vi "Set Stop Trigger (Log Indefinitely).vi"(8 "error in (no error)":errorcluster, 11 "Data Logging Specification Ref in":T1) -> (0 "error out":errorcluster, 3 "Data Logging Specification Ref out":T1)   [LabVIEW 2020, in "NI_VS Data Logging API.lvlib"]
doc: "Specifies a trigger condition on which to stop logging data. You also can specify whether to continue logging channel data for a set period of time after the trigger condition occurs.\n\nYou must manually select the polymorphic instance to use."
uses:
  <vilib>/NI VeriStand/Execution/DataLogging/NI_VS Data Logging API.lvlib
  <vilib>/NI VeriStand/Execution/DataLogging/DataLoggingSpecification Ref.ctl
  NationalInstruments.VeriStand.ClientAPI
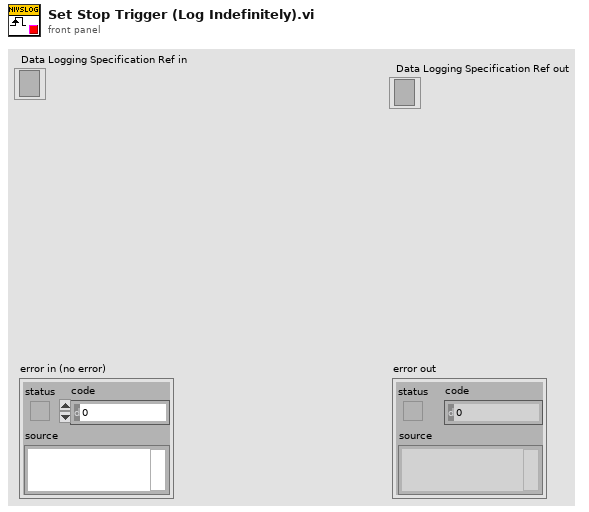
[diagram p1: front panel]
types:
  T1 = typedef "NI_VS Data Logging API.lvlib/DataLoggingSpecification Ref.ctl" = refnum<k24>
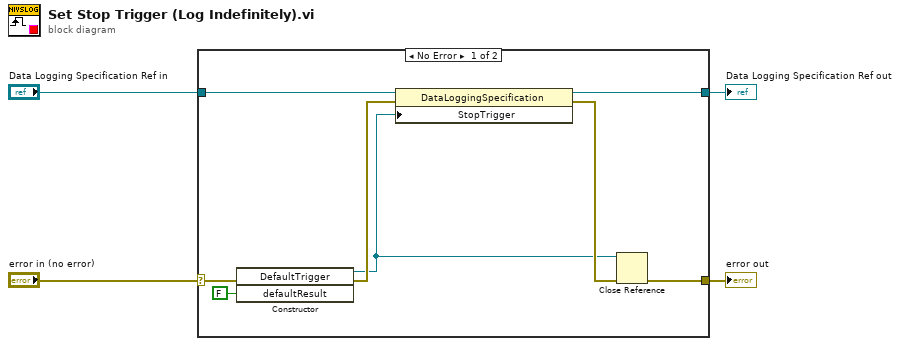
[diagram p0: block diagram]
diagram:
  n1 = case shown="No Error" "error in (no error)" {
    selector: "error in (no error)" -> [w9 w14]
    tunnel: "Data Logging Specification Ref in" -> [w10 w13]
    tunnel: [w6 w13] -> w3
    tunnel: [w5 w14] -> w2
    frame No Error {
      n2 = constructor class="DefaultTrigger"(error in=w9, "defaultResult"=FALSE) -> (reference out=w8:refnum<k24>, error out=w12:errorcluster)  [unwired: 2 in, 2 out]
      n3 = property class="DataLoggingSpecification"(reference=w10, error in=w12, "StopTrigger"=w8) -> (reference out=w6:T1, error out=w11:errorcluster)
      n4 = Close Reference(reference=w8, error in (no error)=w11) -> (error out=w5:errorcluster)
    }
    frame Error {
    }
  }
  "error out" <- w2
  "Data Logging Specification Ref out" <- w3
